vi "Search for roboRIO.vi"(8 "error in (no error)":errorcluster) -> (0 "error out":errorcluster, 3 "roboRIO Connection Information":T1)   [LabVIEW 2018, in "Personalities Tool.lvlib"]
uses:
  Personalities Tool.lvlib
  Controls/roboRIO Connection Information.ctl
  Controls/Personality Type.ctl
panel:
  in  "IP Address 2":string
  in  "SN 2":string
  in  "Commit":bool
  in  "roboRIO found? 2":bool
  in  "roboRIO personality 2":string
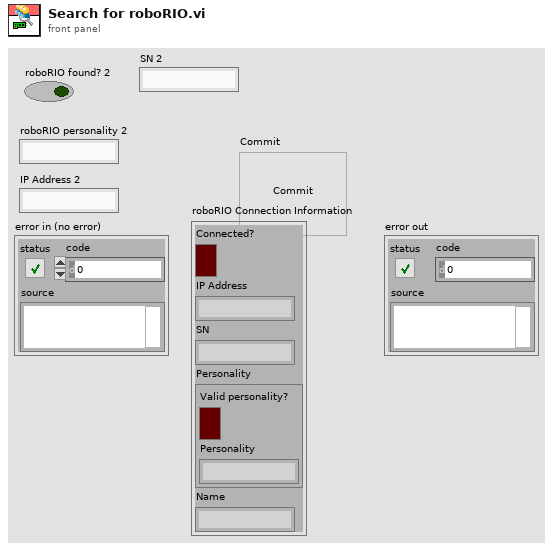
[diagram p1: front panel]
types:
  T1 = typedef "Personalities Tool.lvlib/roboRIO Connection Information.ctl" = cluster{"Connected?":bool, "IP Address":string, "SN":string, "Personality":T2, "Name":string}
  T2 = typedef "Personalities Tool.lvlib/Personality Type.ctl" = cluster{"Valid personality?":bool, "Personality":string}
  T3 = cluster{"Valid personality?":bool, "Personality":string}
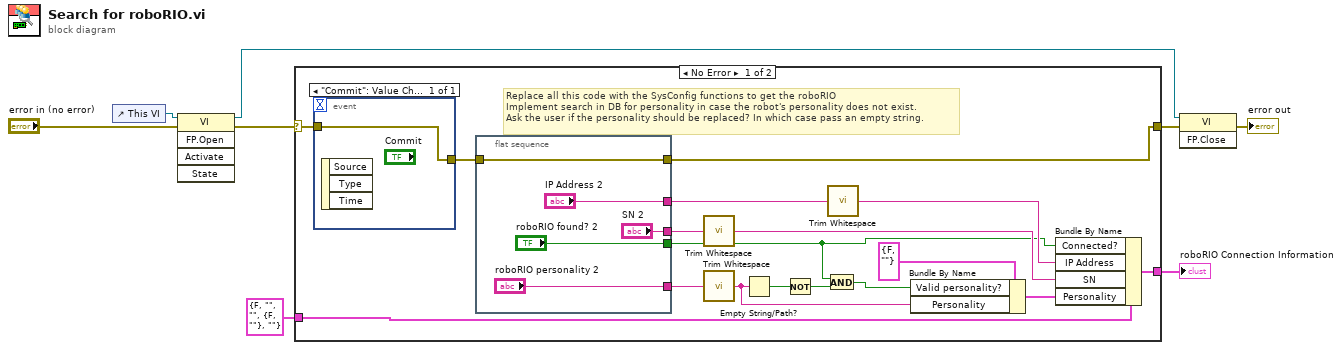
[diagram p0: block diagram]
diagram:
  n1 = control-ref of="This VI"() -> (w6:refnum<vi>)
  n2 = invoke class="VI" method="FP.Open"(reference=w6, error in="error in (no error)") -> (reference out=w3:refnum<vi>, error out=w7:errorcluster)  [unwired: 3 in, 3 out]
  n3 = case shown="No Error" w7 {
    selector: w7 -> [w21 w33]
    tunnel: [w25 w33] -> w4
    tunnel: T1 {"Connected?"=FALSE, "IP Address"="", "SN"="", "Personality"={"Valid personality?"=FALSE, "Personality"=""}, "Name"=""} ("roboRIO Connection Information") -> [w14 w32]
    tunnel: [w13 w32] -> w1
    frame No Error {
      # "Replace all this code with the SysConfig functions to get the roboRIO\nImplement search in DB for personality in case the robot's personality does not exist.\nAsk the user if the personality should be replaced? In which case pass an empty string."
      n4 = event shown="[0] \"Commit\": Value Change" {
        selector: _ -> [_]
        dyn-events: _ -> [_]
        timeout: _ -> [_]
        tunnel: [w31] -> w20
        tunnel: w21 -> [w31]
        event "Commit": Value Change {
          n5 = event-data() -> ()  [unwired: 1 in, 3 out]
        }
      }
      n6 = flat-sequence {
        tunnel: [w30] -> w25
        tunnel: w20 -> [w30]
        tunnel: ["roboRIO found? 2"] -> w9
        tunnel: ["roboRIO personality 2"] -> w24
        tunnel: ["IP Address 2"] -> w23
        tunnel: ["SN 2"] -> w22
        frame #0 {
        }
      }
      n7 = call <vilib>:"Trim Whitespace.vi"("string"=w22) -> ("trimmed string"=w11:string)  [unwired: 1 in]
      n8 = call <vilib>:"Trim Whitespace.vi"("string"=w24) -> ("trimmed string"=w18:string)  [unwired: 1 in]
      n9 = Empty String/Path?(string/path=w18) -> (empty?=w17:bool)
      n10 = Not(x=w17) -> (.not. x?=w16:bool)
      n11 = And(x=w9, y=w16) -> (x .and. y?=w15:bool)
      n12 = call <vilib>:"Trim Whitespace.vi"("string"=w23) -> ("trimmed string"=w10:string)  [unwired: 1 in]
      n13 = Bundle By Name(cluster=T3 {"Valid personality?"=FALSE, "Personality"=""} ("roboRIO personality"), "Valid personality?"=w15, "Personality"=w18) -> (w12:T3)
      n14 = Bundle By Name(cluster=w14, "Connected?"=w9, "IP Address"=w10, "SN"=w11, "Personality"=w12) -> (w13:T1)
    }
    frame Error {
    }
  }
  "roboRIO Connection Information" <- w1
  n15 = invoke class="VI" method="FP.Close"(reference=w3, error in=w4) -> (error out=→"error out":errorcluster)  [unwired: 1 in, 2 out]
